vi "WindToSailLookup.vi"(11 "RelativeWindAngle":dbl) -> (3 "Suggested Sail Setpoints":T1 {"MainSailSuggestion" min=0.0 max=1.0; "JibSailSuggestion" min=0.0 max=1.0})   [LabVIEW 2012]
doc: "Spring 2014\n\nInput: Relative Wind Angles\n\nReturns suggestions for the angle of the main sail and the angle of the jib sail, from a lookup table of wind to sail angles."
uses:
  Data/TypeDefs/Sail Set Suggestions.ctl
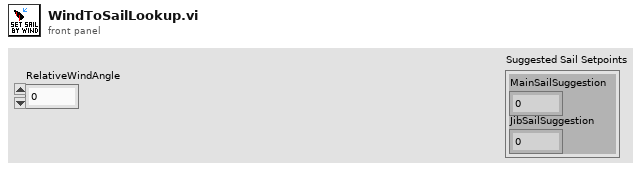
[diagram p1: front panel]
types:
  T1 = typedef "Sail Set Suggestions.ctl" = cluster{"MainSailSuggestion":dbl, "JibSailSuggestion":dbl}
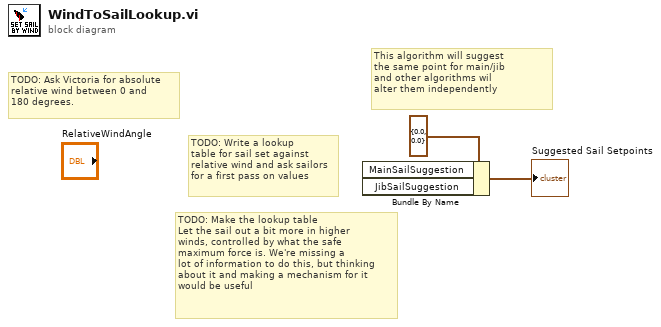
[diagram p0: block diagram]
diagram:
  # "TODO: Make the lookup table\nLet the sail out a bit more in higher\nwinds, controlled by what the safe\nmaximum force is. We're missing a\nlot of information to do this, but thinking\nabout it and making a mechanism for it\nwould be useful"
  # "TODO: Ask Victoria for absolute\nrelative wind between 0 and\n180 degrees."
  # "TODO: Write a lookup\ntable for sail set against\nrelative wind and ask sailors\nfor a first pass on values"
  # "This algorithm will suggest\nthe same point for main/jib\nand other algorithms wil\nalter them independently"
  n1 = Bundle By Name(cluster=T1 {"MainSailSuggestion"=0.0, "JibSailSuggestion"=0.0} ("output cluster")) -> (→"Suggested Sail Setpoints":T1)  [unwired: 2 in]
